vi "Celcius to fahrenheit.vi"() -> ()   [LabVIEW 2016]
panel:
  out "Thermometer":dbl(slide) scale=0.0..100.0
  out "Fahrenheit":dbl
  in  "Celsius":dbl(knob) scale=0.0..10.0
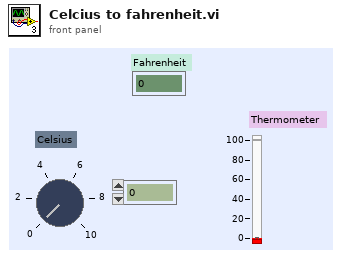
[diagram p1: front panel]
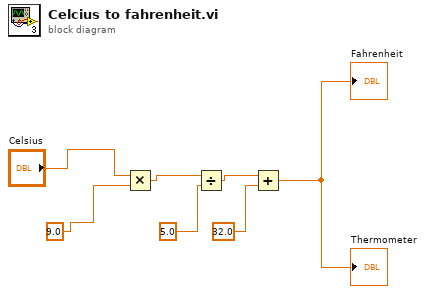
[diagram p0: block diagram]
diagram:
  n1 = Multiply(x="Celsius", y=9.0) -> (x*y=w5:dbl)
  n2 = Divide(x=w5, y=5.0 ("x/y")) -> (x/y=w3:dbl)
  n3 = Add(x=w3, y=32.0) -> (x+y=→"Fahrenheit" →"Thermometer":dbl)
